vi "WPI_CameraAcquire MJPG Loop.vi"(11 "CameraDevRef":T1) -> ()   [LabVIEW 2017]
doc: "This VI acquires the image buffer from the camera MJPG stream at the configured fps rate. It notifies any waiting VIs and allows them to pick up the latest image. This allows the camera and robot vision loop to run at different rates. The 1011, camera is far more efficient using MJPGs, and generally, this is probably the better choice for the camera loop.\n \nThis software is licensed. Open the labview\\readme\\WPI Robotics Library Open Source License.txt file for more information."
uses:
  <vilib>/Rock Robotics/WPI/Camera/WPI_CameraDevRef.ctl
  <vilib>/Rock Robotics/WPI/Camera/WPI_CameraSettings Operations.ctl
  <vilib>/Rock Robotics/WPI/Camera/WPI_CameraSettings Read MJPG.ctl
  <vilib>/Rock Robotics/WPI/Camera/WPI_CameraImageSize.ctl
panel:
  out "connection ID":refnum<k5>
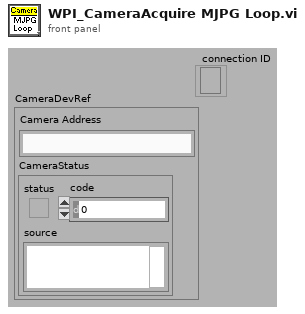
[diagram p1: front panel]
types:
  T1 = typedef "WPI_CameraDevRef.ctl" = cluster{"Camera Address":string, "CameraStatus":errorcluster}
  T2 = typedef "WPI_CameraSettings Operations.ctl" = enum16{"Udate FPS", "Update Compression", "Update Size", "Update White Balance", "Update Brightness", "Update Sharpness", "Update Exposure", "Update Exposure Value", "Update Color Level", "Update Exp Priority", "Update Color Enable", "Update JPG", "Update MJPG", "Read and Clear", "Read", "Init"}
  T3 = typedef "WPI_CameraSettings Read MJPG.ctl" = cluster{"fps":i32, "compression":i32, "Image Size":T4, "Config Shown":bool}
  T4 = typedef "WPI_CameraImageSize.ctl" = enum16{"640x480", "320x240", "160x120", "Custom"}
  T5 = typedef "WPI_CameraSettings Control.ctl" = cluster{"FPS":i32, "Compression":i32, "Size":i32, "White Balance":i32, "Brightness":i32, "Sharpness":i32, "Exposure":i32, "Color Level":i32, "Exposure Priority":i32, "Color Enable":i32, "JPG Loop":i32, "MJPG Loop":i32, "Exposure Value":i32}
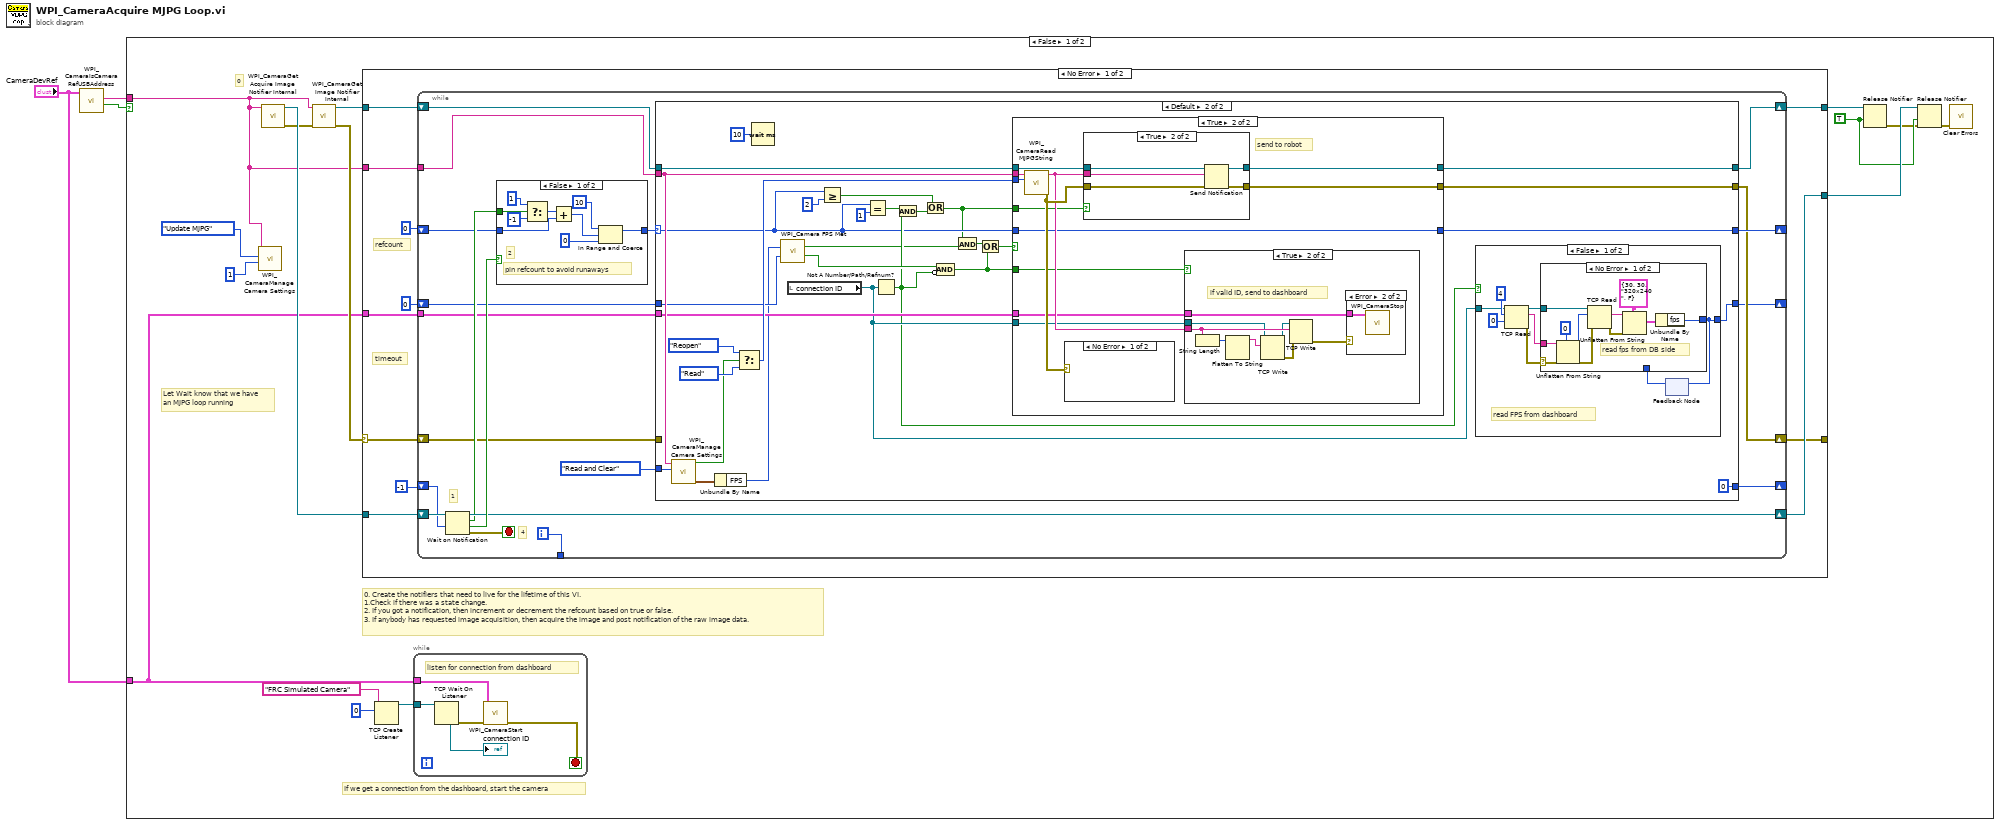
[diagram p0: block diagram]
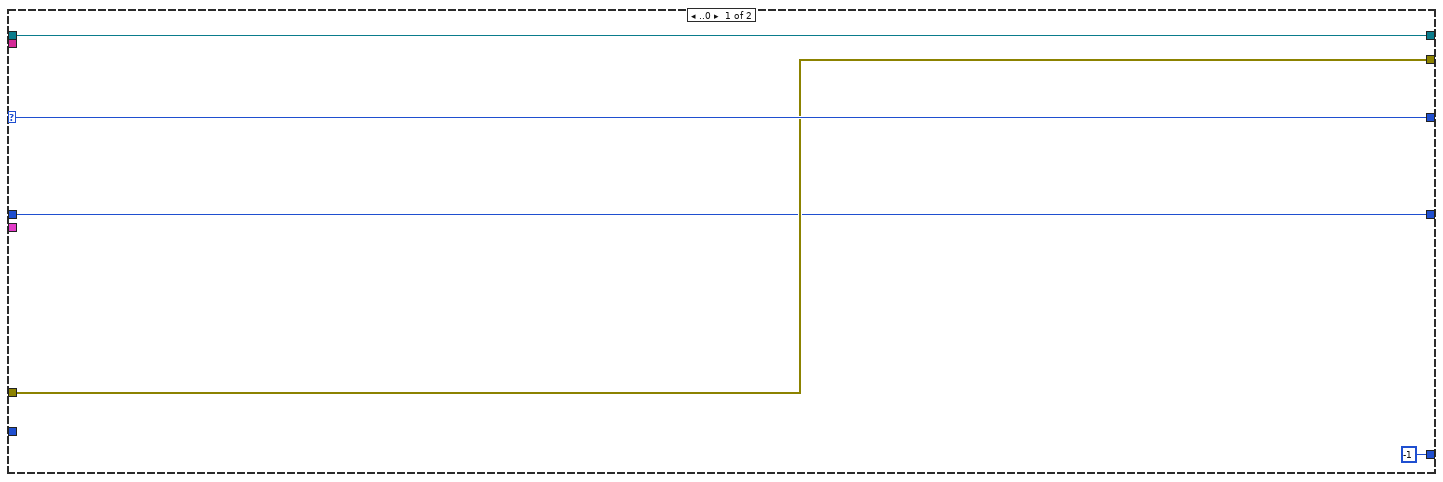
[diagram p2: hidden frame]
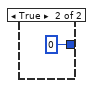
[diagram p4: hidden frame]
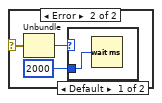
[diagram p9: hidden frame]
diagram:
  n1 = call <vilib>:"WPI_CameraIsCameraRefUSBAddress.vi"("CameraDevRef"="CameraDevRef") -> ("USB?"=w1:bool, "Camera Address Out"=w2:string)  [unwired: 7 in, 2 out]
  n2 = case shown="False" w1 {
    tunnel: "CameraDevRef" -> [w5 _]
    tunnel: w2 -> [w4 _]
    frame False {
      w16 = TRUE ("force destroy? (F)")
      # "If we get a connection from the dashboard, start the camera"
      # "Let Wait know that we have\nan MJPG loop running"
      # "0"
      # "0. Create the notifiers that need to live for the lifetime of this VI. \n1.Check if there was a state change.\n2. If you got a notification, then increment or decrement the refcount based on true or false.\n3. If anybody has requested image acquisition, then acquire the image and post notification of the raw image data."
      n3 = call <vilib>:"WPI_CameraManage Camera Settings.vi"("Value"=1, "Operation"=WPI_CameraSettings_Operations."Update MJPG", "Camera IP"=w4) -> ()  [unwired: 7 in, 2 out]
      n4 = call <vilib>:"WPI_CameraGet Acquire Image Notifier Internal.vi"("Camera Address"=w4) -> ("error out"=w12:errorcluster, "Acquire Image Notifier"=w13:refnum<notifier>)  [unwired: 1 in, 8 out]
      n5 = call <vilib>:"WPI_CameraGet Image Notifier Internal.vi"("error in (no error)"=w12, "Camera Address"=w4) -> ("error out"=w15:errorcluster, "Image Notifier"=w17:refnum<notifier>)  [unwired: 8 out]
      n6 = case shown="No Error" w15 {
        selector: w15 -> [w28 w159]
        tunnel: w4 -> [w35 _]
        tunnel: w13 -> [w34 w157]
        tunnel: w17 -> [w32 w158]
        tunnel: [w30 w158] -> w19
        tunnel: [w29 w157] -> w18
        tunnel: [w27 w159] -> _
        tunnel: w5 -> [w26 _]
        frame No Error {
          # "timeout"
          # "refcount"
          n7 = while {
            shift-right: [w53] -> w29
            shift-left: w34 -> [w55]
            tunnel: w35 -> [w50]
            shift-right: [w42] -> _
            shift-left: 0 -> [w51]
            shift-right: [w48] -> w30
            shift-left: w32 -> [w49]
            shift-right: [w46] -> _
            shift-left: -1 -> [w47]
            shift-right: [w41] -> w27
            shift-left: w28 -> [w44]
            tunnel: [w39] -> _
            tunnel: w26 -> [w38]
            shift-right: [w37] -> _
            shift-left: 0 ("fps") -> [w36]
            i -> [w39]
            stop <- w45 stop-if-true
            # "4"
            # "1"
            n8 = Wait on Notification(notifier=w55, timeout in ms (-1)=w47) -> (notifier out=w53:refnum<notifier>, notification=w52:bool, timed out?=w54:bool, error out=w45:errorcluster)  [unwired: 1 in, 1 out]
            n9 = case shown="False" w54 {
              tunnel: w52 -> [w155 _]
              tunnel: w51 -> [w151 w156]
              tunnel: [w147 w156] -> w43
              frame False {
                # "pin refcount to avoid runaways"
                # "2"
                n10 = Select(t=1, s=w155, f=-1) -> (s? t:f=w152:i32)
                n11 = Add(x=w152, y=w151) -> (x+y=w148:i32)
                n12 = In Range and Coerce(upper limit=10, x=w148, lower limit=0) -> (coerced(x)=w147:i32)  [unwired: 1 out]
              }
              frame True {
              }
            }
            n13 = case shown="Default" w43 {
              selector: w43 -> [w59 w65]
              tunnel: w50 -> [_ w81]
              tunnel: w49 -> [w60 w91]
              tunnel: [w60 w90] -> w48
              tunnel: [-1 0] -> w46
              tunnel: w44 -> [w57 _]
              tunnel: [w59 w75] -> w42
              tunnel: [w57 w88] -> w41
              tunnel: WPI_CameraSettings_Operations."Read and Clear" ("Operation") -> [_ w82]
              tunnel: w38 -> [_ w80]
              tunnel: [w56 w74] -> w37
              tunnel: w36 -> [w56 w78]
              frame ..0 {
              }
              frame Default {
                n14 = call <vilib>:"WPI_CameraManage Camera Settings.vi"("Operation"=w82, "Camera IP"=w81) -> ("Values"=w83:T5, "Changed"=w84:bool)  [unwired: 8 in]
                n15 = Unbundle By Name(w83) -> ("FPS"=w77:i32)
                n16 = Select(t=enum16{"Read", "Reopen", "Close"}."Reopen" ("Operation"), s=w84, f=enum16{"Read", "Reopen", "Close"}."Read" ("Operation")) -> (s? t:f=w85:enum16{"Read", "Reopen", "Close"})
                n17 = Wait (ms)(milliseconds to wait=u32 10) -> ()  [unwired: 1 out]
                n18 = call <vilib>:"WPI_Camera FPS Met.vi"("robot fps"=w77, "dashboard fps"=w78) -> ("robot fps met?"=w66:bool, "dashboard fps met?"=w71:bool)  [unwired: 12 in]
                n19 = local read "connection ID"() -> (w73:refnum<k5>)
                n20 = Greater Or Equal?(x=w65, y=2) -> (x >= y?=w62:bool)
                n21 = Equal?(x=w65, y=1) -> (x = y?=w68:bool)
                n22 = Not A Number/Path/Refnum?(number/path/refnum=w73) -> (NaN/Path/Refnum?=w69:bool)
                n23 = And(x=w68, y=w69) -> (x .and. y?=w63:bool)
                n24 = Or(x=w62, y=w63) -> (x .or. y?=w61:bool)
                n25 = Compound Arithmetic op=AND(w71, invert w69) -> (w72:bool)
                n26 = And(x=w61, y=w66) -> (x .and. y?=w67:bool)
                n27 = Or(x=w67, y=w72) -> (x .or. y?=w76:bool)
                n28 = case shown="True" w76 {
                  tunnel: w91 -> [w114 w126]
                  tunnel: [w114 w125] -> w90
                  tunnel: [_ w124] -> w88
                  tunnel: w85 -> [_ w123]
                  tunnel: w81 -> [_ w122]
                  tunnel: w65 -> [w113 w117]
                  tunnel: w73 -> [_ w119]
                  tunnel: w80 -> [_ w118]
                  tunnel: [w113 w117] -> w75
                  tunnel: w72 -> [_ w116]
                  tunnel: w61 -> [_ w115]
                  frame False {
                  }
                  frame True {
                    # "send to robot"
                    n29 = call <vilib>:"WPI_CameraRead MJPGString.vi"("Operation"=w123, "address"=w122) -> ("error out"=w121:errorcluster, "Raw Image Data"=w120:string)  [unwired: 8 in]
                    n30 = case shown="No Error" w121 {
                      selector: w121 -> [_ w145]
                      frame No Error {
                      }
                      frame Error {
                        n31 = Unbundle(w145) -> ("code"=w144:i32)  [unwired: 2 out]
                        n32 = case shown="Default" w144 {
                          tunnel: u32 2000 ("milliseconds to wait") -> [w146 _]
                          frame Default {
                            n33 = Wait (ms)(milliseconds to wait=w146) -> ()  [unwired: 1 out]
                          }
                          frame 56 {
                          }
                        }
                      }
                    }
                    n34 = case shown="True" w115 {
                      tunnel: w126 -> [w137 w142]
                      tunnel: [w137 w141] -> w125
                      tunnel: [w136 w140] -> w124
                      tunnel: w121 -> [w136 w139]
                      tunnel: w120 -> [_ w138]
                      frame False {
                      }
                      frame True {
                        n35 = Send Notification(notification=w138, notifier=w142, error in (no error)=w139) -> (notifier out=w141:refnum<notifier>, error out=w140:errorcluster)
                      }
                    }
                    n36 = case shown="True" w116 {
                      tunnel: w120 -> [_ w134]
                      tunnel: w119 -> [_ w131]
                      tunnel: w118 -> [_ w127]
                      frame False {
                      }
                      frame True {
                        # "if valid ID, send to dashboard"
                        n37 = String Length(string=w134) -> (length=w133:i32)
                        n38 = Flatten To String(anything=w133) -> (data string=w132:string)  [unwired: 3 in, 2 out]
                        n39 = TCP Write(connection ID=w131, data in=w132) -> (connection ID out=w128:refnum<k5>, error out=w130:errorcluster)  [unwired: 2 in, 1 out]
                        n40 = TCP Write(connection ID=w128, data in=w134, error in (no error)=w130) -> (error out=w129:errorcluster)  [unwired: 1 in, 2 out]
                        n41 = case shown="Error" w129 {
                          tunnel: w127 -> [_ w135]
                          frame No Error {
                          }
                          frame Error {
                            n42 = call <vilib>:"WPI_CameraStop.vi"("CameraDevRef"=w135) -> ()  [unwired: 1 in, 10 out]
                          }
                        }
                      }
                    }
                  }
                }
                n43 = case shown="False" w69 {
                  tunnel: [w94 0 ("fps")] -> w74
                  tunnel: w73 -> [w92 _]
                  frame False {
                    # "read FPS from dashboard"
                    n44 = TCP Read(connection ID=w92, bytes to read=4, 9:0 ("timeout ms (25000)")) -> (connection ID out=w96:refnum<k5>, data out=w97:string, error out=w95:errorcluster)  [unwired: 2 in]
                    n45 = feedback #1() -> (w93:i32)  [unwired: 1 in]
                    n46 = case shown="No Error" w95 {
                      selector: w95 -> [w101 _]
                      tunnel: w97 -> [w109 _]
                      tunnel: w96 -> [w107 _]
                      tunnel: [w100 w111] -> w94
                      tunnel: w93 -> [_ w111]
                      frame No Error {
                        # "read fps from DB side"
                        n47 = Unflatten From String(type=0 ("bytes to read"), binary string=w109, error in (no error)=w101) -> (value=w106:i32, error out=w108:errorcluster)  [unwired: 2 in, 1 out]
                        n48 = TCP Read(connection ID=w107, bytes to read=w106, error in (no error)=w108) -> (data out=w105:string, error out=w104:errorcluster)  [unwired: 1 in, 2 out]
                        n49 = Unflatten From String(type=T3 {"fps"=30, "compression"=30, "Image Size"=enum."320x240", "Config Shown"=FALSE} ("Camera Settings"), binary string=w105, error in (no error)=w104) -> (value=w102:T3)  [unwired: 2 in, 2 out]
                        n50 = Unbundle By Name(w102) -> ("fps"=w100:i32)
                      }
                      frame Error {
                      }
                    }
                    n51 = feedback-in #1(w94) -> ()
                  }
                  frame True {
                  }
                }
              }
            }
          }
        }
        frame Error {
        }
      }
      n52 = TCP Create Listener(10:u16 0 ("port"), 11:"FRC Simulated Camera" ("service name")) -> (3:w8:refnum<k5>)  [unwired: 3 in, 2 out]
      n53 = while {
        tunnel: w8 -> [w24]
        tunnel: w5 -> [w20]
        stop <- w21 stop-if-true
        # "listen for connection from dashboard"
        n54 = TCP Wait On Listener(11:w24) -> (0:w22:errorcluster, 4:→"connection ID":refnum<k5>)  [unwired: 3 in, 3 out]
        n55 = call <vilib>:"WPI_CameraStart.vi"("error in (no error)"=w22, "CameraDevRef"=w20) -> ("error out"=w21:errorcluster)  [unwired: 9 out]
      }
      n56 = Release Notifier(notifier=w19, force destroy? (F)=w16) -> (error out=w11:errorcluster)  [unwired: 1 in, 2 out]
      n57 = Release Notifier(notifier=w18, force destroy? (F)=w16, error in (no error)=w11) -> (error out=w14:errorcluster)  [unwired: 2 out]
      n58 = call <vilib>:"Clear Errors.vi"("error in (no error)"=w14) -> ()  [unwired: 1 in, 6 out]
    }
    frame True {
    }
  }
